vi "String to time.vi"(3 "Строка со временем":string) -> (0 "Время в секундах":dbl, 1 "Время всего процесса":timestamp=timestamp(-10799.315441346698 s since 1904-01-01) format="%<%H:%M:%S>T")   [LabVIEW 2016]
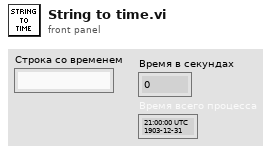
[diagram p1: front panel]
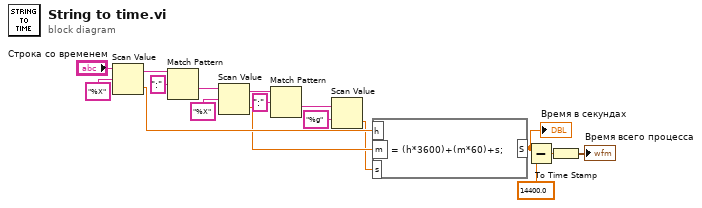
[diagram p0: block diagram]
diagram:
  n1 = Scan Value(string="Строка со временем", format string="%X" ("time format string (%c)")) -> (output string=w16:string, value=w12:dbl)  [unwired: 1 in]
  n2 = Match Pattern(string=w16, regular expression=":") -> (after substring=w13:string)  [unwired: 1 in, 3 out]
  n3 = Scan Value(string=w13, format string="%X" ("time format string (%c)")) -> (output string=w8:string, value=w11:dbl)  [unwired: 1 in]
  n4 = Match Pattern(string=w8, regular expression=":") -> (after substring=w9:string)  [unwired: 1 in, 3 out]
  n5 = Scan Value(string=w9, format string="%g") -> (value=w7:dbl)  [unwired: 1 in, 1 out]
  n6 = formula code="S = (h*3600)+(m*60)+s;"("h"=w12, "m"=w11, "s"=w7) -> ("S"=w1:dbl)
  "Время в секундах" <- w1
  n7 = Subtract(x=w1, y=14400.0) -> (x-y=w4:dbl)
  n8 = To Time Stamp(1:w4) -> (0:→"Время всего процесса":timestamp)
